vi "Add Tests.vi"(8 "error in (no error)":errorcluster, 10 "Test Cases":refnum<class "Test Case.lvclass">[](array[class]), 11 "ResultTree in":refnum<class "ResultTree.lvclass">) -> (0 "error out":errorcluster, 3 "ResultTree out":refnum<class "ResultTree.lvclass">)   [LabVIEW 2017, in "ResultTree.lvclass"]
doc: "Adds the specified list of test cases to the tree. The hierarchy is determined from the qualified names."
uses:
  ResultTree.lvclass
  Test Case/Test Case.lvclass
  ResultTree.lvclass/ResultTree.ctl
  Test Case/Test Case.lvclass/Test Case.ctl
  Test Case/Get Qualified Name.vi
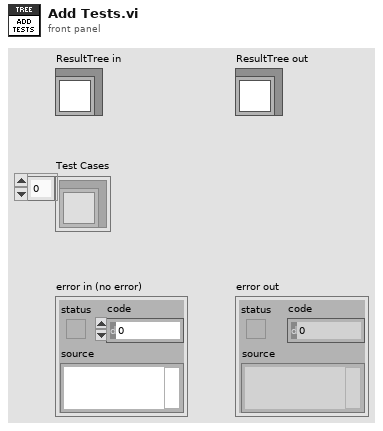
[diagram p1: front panel]
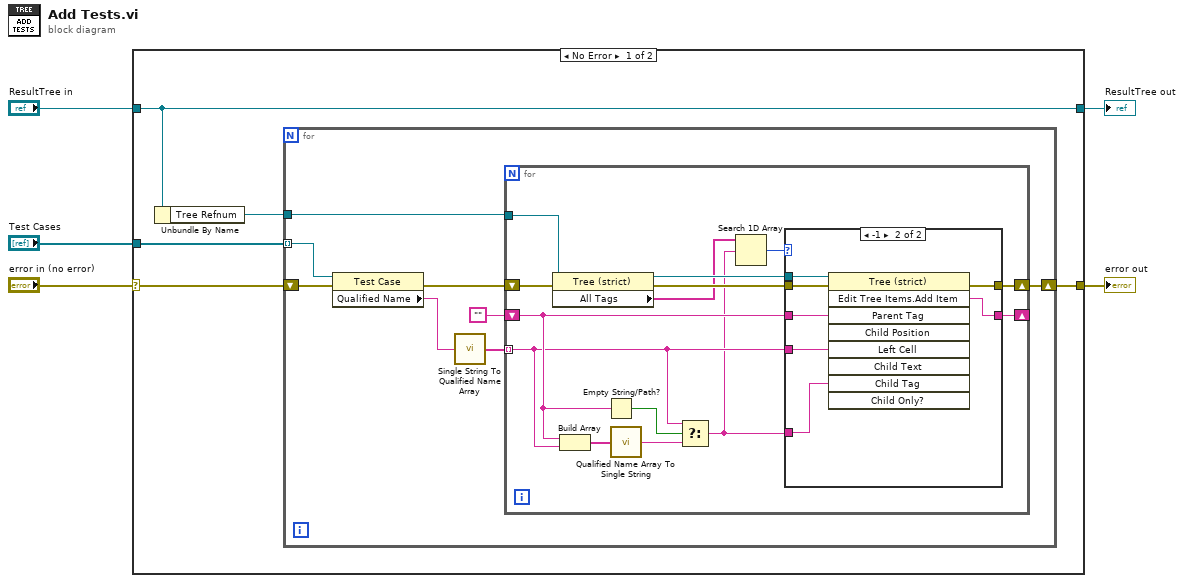
[diagram p0: block diagram]
diagram:
  n1 = case shown="No Error" "error in (no error)" {
    selector: "error in (no error)" -> [w10 w43]
    tunnel: [w9 w43] -> w4
    tunnel: [w8 w42] -> w2
    tunnel: "ResultTree in" -> [w8 w42]
    tunnel: "Test Cases" -> [w6 _]
    frame No Error {
      n2 = Unbundle By Name(w8) -> ("Tree Refnum"=w7:refnum<vi>)
      n3 = for {
        tunnel: w7 -> [w16]
        tunnel: w6 -> [w14] mode=indexing
        shift-right: [w17] -> w9
        shift-left: w10 -> [w18]
        n4 = property class="Test Case"(reference=w14, error in=w18) -> (error out=w15:errorcluster, "Qualified Name"=w13:string)  [unwired: 1 out]
        n5 = call <vilib>:"Single String To Qualified Name Array.vi"("Fully Qualified String"=w13) -> ("Fully Qualified Array"=w12:string[])
        n6 = for {
          tunnel: w16 -> [w29]
          shift-right: [w31] -> w17
          shift-left: w15 -> [w32]
          tunnel: w12 -> [w20] mode=indexing
          shift-right: [w25] -> _
          shift-left: "" -> [w21]
          n7 = property class="Tree (strict)"(reference=w29, error in=w32) -> (reference out=w28:refnum<vi>, error out=w30:errorcluster, "All Tags"=w27:string[])
          n8 = Build Array(w21, w20) -> (w24:string[])
          n9 = Empty String/Path?(string/path=w21) -> (empty?=w22:bool)
          n10 = call <vilib>:"Qualified Name Array To Single String.vi"("Fully Qualified Array"=w24) -> ("Fully Qualified String"=w23:string)
          n11 = Select(t=w20, s=w22, f=w23) -> (s? t:f=w19:string)
          n12 = Search 1D Array(1D array=w27, element=w19) -> (index of element=w26:i32)  [unwired: 1 in]
          n13 = case shown="-1" w26 {
            tunnel: [w34 w41] -> w31
            tunnel: w30 -> [w34 w40]
            tunnel: w28 -> [_ w39]
            tunnel: w21 -> [_ w38]
            tunnel: [w33 w37] -> w25
            tunnel: w19 -> [w33 w36]
            tunnel: w20 -> [_ w35]
            frame Default {
            }
            frame -1 {
              n14 = invoke class="Tree (strict)" method="Edit Tree Items.Add Item"(reference=w39, error in=w40, "Parent Tag"=w38, "Left Cell"=w35, "Child Tag"=w36) -> (error out=w41:errorcluster, "Edit Tree Items:Add Item"=w37:string)  [unwired: 4 in, 7 out]
            }
          }
        }
      }
    }
    frame Error {
    }
  }
  "error out" <- w4
  "ResultTree out" <- w2
